vi "AgNA_Channel Measurement Fetch Formatted.vi"(8 "error in (no error)":errorcluster {"code" format="%.0x"}, 9 "RetValBufferSize":i32=2048, 10 "RepCapIdentifier":string, 11 "instrument handle":refnum<k15>) -> (0 "error out":errorcluster {"code" format="%.0x"}, 1 "RetValActualSize":i32, 2 "RetVal":dbl[](array[numeric]) format="%.2p", 3 "instrument handle out":refnum<k15>)   [LabVIEW 2015]
uses:
  <instrlib>/Agilent NA/Agilent NA.lvlib
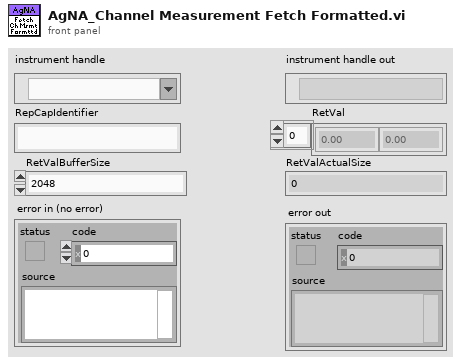
[diagram p1: front panel]
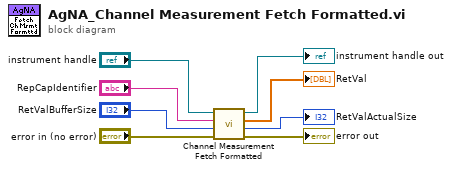
[diagram p0: block diagram]
diagram:
  n1 = call <instrlib>:"Channel Measurement Fetch Formatted.vi"("error in (no error)"="error in (no error)", "RetValBufferSize"="RetValBufferSize", "RepCapIdentifier"="RepCapIdentifier", "instrument handle"="instrument handle") -> ("error out"=→"error out":errorcluster, "RetValActualSize"=→"RetValActualSize":i32, "RetVal"=→"RetVal":dbl[], "instrument handle out"=→"instrument handle out":refnum<k15>)  [unwired: 4 in]
